vi "Auto Stack.vi"(9 "Stop Lift":bool, 10 "Reset Tote Count":bool, 11 "Use Auto Stack":bool) -> (3 "Tote Count":dbl)   [LabVIEW 2014]
uses:
  TypeDefs/SRE Enum.ctl
  Support Code/Robot Global Data.vi
panel:
  out "State Last":T1(ring)=enum."Stopped"
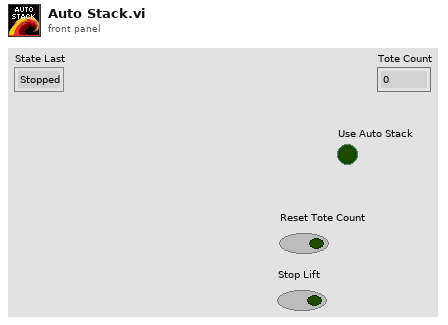
[diagram p1: front panel]
types:
  T1 = enum16{"Wait", "Lift Down", "Lift Up", "Align Tote", "Nothing", "Stopped"}
  T2 = enum16{"Wait", "Lift Down", "Lift Up", "Align Tote", "Nothing"}
  T3 = typedef "SRE Enum.ctl" = enum16{"Start", "Run", "End"}
  T4 = enum16{"High", "Middle", "Low", "Really Low", "Stopped"}
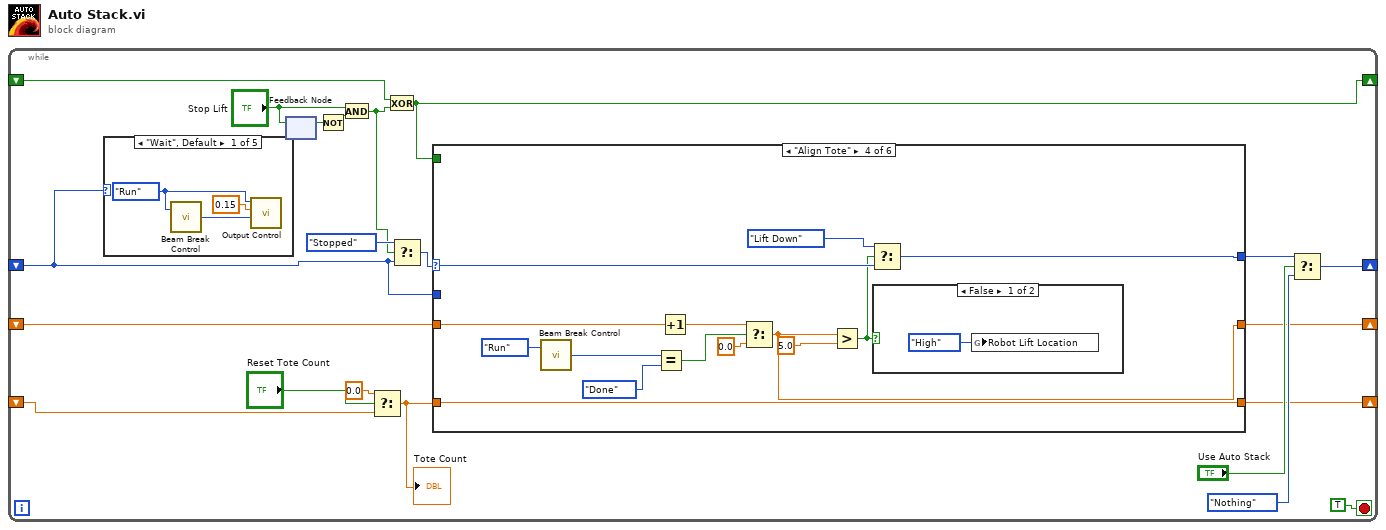
[diagram p0: block diagram]
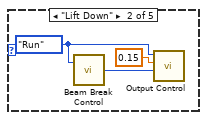
[diagram p2: hidden frame]
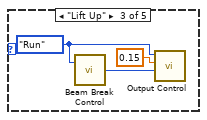
[diagram p3: hidden frame]
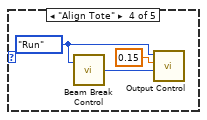
[diagram p4: hidden frame]
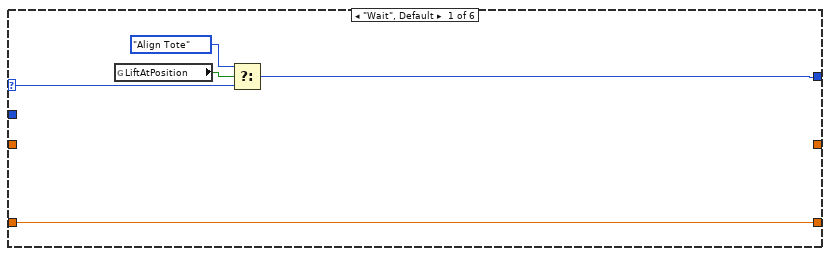
[diagram p6: hidden frame]
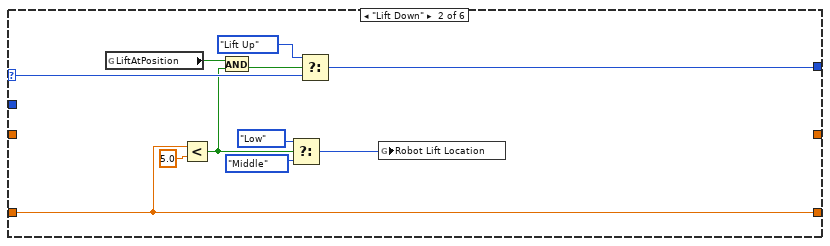
[diagram p7: hidden frame]
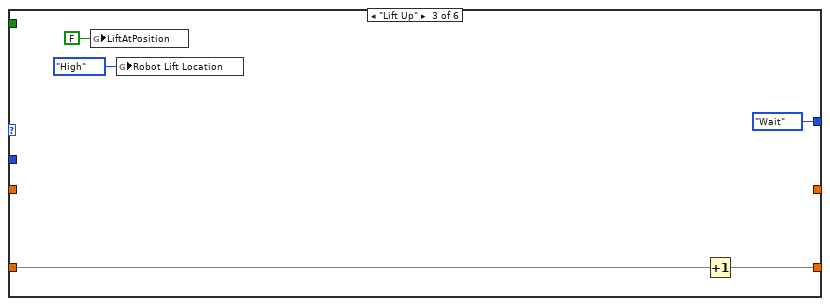
[diagram p8: hidden frame]
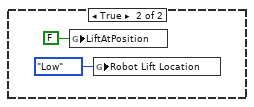
[diagram p9: hidden frame]
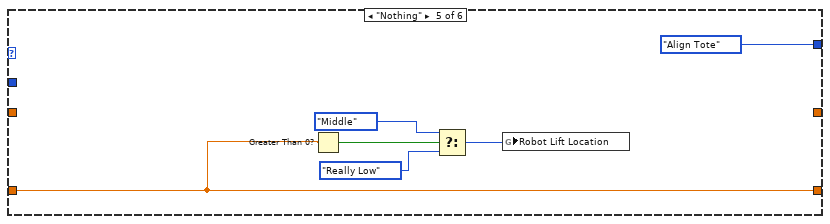
[diagram p10: hidden frame]
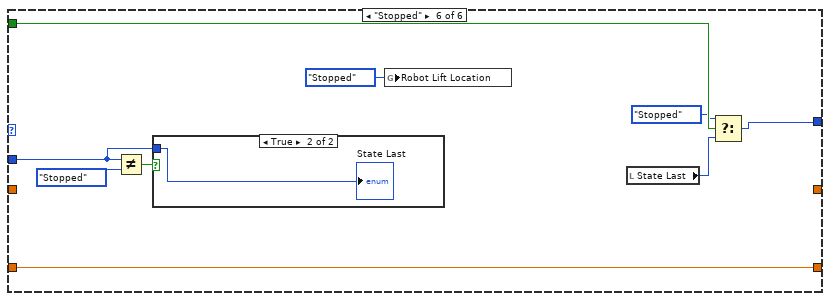
[diagram p11: hidden frame]
diagram:
  n1 = while {
    shift-right: [w20] -> _
    shift-left: _ -> [w9]
    shift-right: [w16] -> _
    shift-left: _ -> [w13]
    shift-right: [w11] -> _
    shift-left: _ -> [w10]
    shift-right: [w2] -> _
    shift-left: _ -> [w3]
    stop <- TRUE stop-if-true
    n2 = case shown="\"Wait\", Default" w9 {
      frame "Wait", Default {
        w23 = SRE_Enum."Run" ("SRE")
        n3 = call "Beam Break Control.vi"("SRE"=w23) -> ("Enum"=w24:enum16{"In", "Out", "Done"})  [unwired: 2 in]
        n4 = call "Output Control.vi"("Direction"=w24, "Power"=0.15, "Mode"=w23) -> ()  [unwired: 9 in]
      }
      frame "Lift Down" {
        w26 = SRE_Enum."Run" ("SRE")
        n5 = call "Beam Break Control.vi"("SRE"=w26) -> ("Enum"=w27:enum16{"In", "Out", "Done"})  [unwired: 2 in]
        n6 = call "Output Control.vi"("Direction"=w27, "Power"=0.15, "Mode"=w26) -> ()  [unwired: 9 in]
      }
      frame "Lift Up" {
        w29 = SRE_Enum."Run" ("SRE")
        n7 = call "Beam Break Control.vi"("SRE"=w29) -> ("Enum"=w30:enum16{"In", "Out", "Done"})  [unwired: 2 in]
        n8 = call "Output Control.vi"("Direction"=w30, "Power"=0.15, "Mode"=w29) -> ()  [unwired: 9 in]
      }
      frame "Align Tote" {
        w32 = SRE_Enum."Run" ("SRE")
        n9 = call "Beam Break Control.vi"("SRE"=w32) -> ("Enum"=w33:enum16{"In", "Out", "Done"})  [unwired: 2 in]
        n10 = call "Output Control.vi"("Direction"=w33, "Power"=0.15, "Mode"=w32) -> ()  [unwired: 9 in]
      }
      frame "Nothing" {
      }
    }
    n11 = feedback-in #1("Stop Lift") -> ()
    n12 = feedback #1() -> (w6:bool)  [unwired: 1 in]
    n13 = Not(x=w6) -> (.not. x?=w5:bool)
    n14 = And(x="Stop Lift", y=w5) -> (x .and. y?=w1:bool)
    n15 = Select(t=0.0, s="Reset Tote Count", f=w13) -> (s? t:f=w12:dbl)
    "Tote Count" <- w12
    n16 = Exclusive Or(1:w1, 2:w3) -> (0:w2:bool)
    n17 = Select(t=T1."Stopped", s=w1, f=w9) -> (s? t:f=w7:T1)
    n18 = case shown="\"Align Tote\"" w7 {
      selector: w7 -> [w38 w49 _ w68 _ _]
      tunnel: [w36 w47 T2."Wait" ("t") w66 T2."Align Tote" ("Auto Stacker State") w78] -> w17
      tunnel: w12 -> [w35 w44 w54 w65 w76 w86]
      tunnel: [w35 w44 w52 w65 w76 w86] -> w16
      tunnel: [_ _ _ w55 _ _] -> w11
      tunnel: w10 -> [_ _ _ w60 _ _]
      tunnel: w2 -> [_ _ _ _ _ w81]
      tunnel: w9 -> [_ _ _ _ _ w82]
      frame "Wait", Default {
        n19 = global read "Robot Global Data.vi" "LiftAtPosition"() -> (w34:bool)
        n20 = Select(t=T2."Align Tote", s=w34, f=w38) -> (s? t:f=w36:T1)
      }
      frame "Lift Down" {
        n21 = global read "Robot Global Data.vi" "LiftAtPosition"() -> (w45:bool)
        n22 = Less?(x=w44, y=5.0) -> (x < y?=w40:bool)
        n23 = And(x=w45, y=w40) -> (x .and. y?=w39:bool)
        n24 = Select(t=enum16{"High", "Middle", "Low"}."Low" ("Robot Lift Location"), s=w40, f=enum16{"High", "Middle", "Low"}."Middle") -> (s? t:f=w41:enum16{"High", "Middle", "Low"})
        n25 = Select(t=T2."Lift Up", s=w39, f=w49) -> (s? t:f=w47:T1)
        n26 = global write "Robot Global Data.vi" "Robot Lift Location"(w41) -> ()
      }
      frame "Lift Up" {
        n27 = global write "Robot Global Data.vi" "LiftAtPosition"(FALSE ("LiftAtPosition")) -> ()
        n28 = global write "Robot Global Data.vi" "Robot Lift Location"(enum16{"High", "Middle", "Low"}."High" ("Robot Lift Location")) -> ()
        n29 = Increment(x=w54) -> (x+1=w52:dbl)
      }
      frame "Align Tote" {
        n30 = call "Beam Break Control.vi"("SRE"=SRE_Enum."Run") -> ("Enum"=w63:enum16{"In", "Out", "Done"})  [unwired: 2 in]
        n31 = Equal?(x=w63, y=enum16{"In", "Out", "Done"}."Done") -> (x = y?=w57:bool)
        n32 = Increment(x=w60) -> (x+1=w59:dbl)
        n33 = Select(t=w59, s=w57, f=0.0) -> (s? t:f=w55:dbl)
        n34 = Greater?(x=w55, y=5.0) -> (0:w56:bool)
        n35 = Select(t=T2."Lift Down", s=w56, f=w68) -> (s? t:f=w66:T1)
        n36 = case shown="False" w56 {
          frame False {
            n37 = global write "Robot Global Data.vi" "Robot Lift Location"(enum16{"High", "Middle", "Low"}."High" ("Robot Lift Location")) -> ()
          }
          frame True {
            n38 = global write "Robot Global Data.vi" "LiftAtPosition"(FALSE ("LiftAtPosition")) -> ()
            n39 = global write "Robot Global Data.vi" "Robot Lift Location"(enum16{"High", "Middle", "Low"}."Low" ("Robot Lift Location")) -> ()
          }
        }
      }
      frame "Nothing" {
        n40 = Greater Than 0?(x=w76) -> (x > 0?=w75:bool)
        n41 = Select(t=enum16{"High", "Middle", "Low", "Really Low"}."Middle" ("Robot Lift Location"), s=w75, f=enum16{"High", "Middle", "Low", "Really Low"}."Really Low" ("Robot Lift Location")) -> (s? t:f=w72:enum16{"High", "Middle", "Low", "Really Low"})
        n42 = global write "Robot Global Data.vi" "Robot Lift Location"(w72) -> ()
      }
      frame "Stopped" {
        n43 = Not Equal?(x=w82, y=T1."Stopped") -> (x != y?=w83:bool)
        n44 = case shown="True" w83 {
          tunnel: w82 -> [_ w87]
          frame False {
          }
          frame True {
            "State Last" <- w87
          }
        }
        n45 = global write "Robot Global Data.vi" "Robot Lift Location"(T4."Stopped" ("Robot Lift Location")) -> ()
        n46 = local read "State Last"() -> (w79:T1)
        n47 = Select(t=T1."Stopped" ("y"), s=w81, f=w79) -> (s? t:f=w78:T1)
      }
    }
    n48 = Select(t=w17, s="Use Auto Stack", f=T2."Nothing" ("Auto Stacker State")) -> (s? t:f=w20:T1)
  }
